vi "StopTask.vi"(8 "error in (no error)":errorcluster, 11 "NI_DAQmx(Linear) in":refnum<class "NI_DAQmx(Linear).lvclass">) -> (0 "error out":errorcluster, 3 "NI_DAQmx(Linear) out":refnum<class "NI_DAQmx(Linear).lvclass">)   [LabVIEW 2025, in "NI_DAQmx(Linear).lvclass"]
uses:
  NI_DAQmx(Linear).lvclass
  NI_DAQmx(Linear).lvclass/NI_DAQmx(Linear).ctl
  Read task.vi
  DAQ_Abstr/Task_Type/Linear_Task/Linear_Task/Linear_Task.lvclass
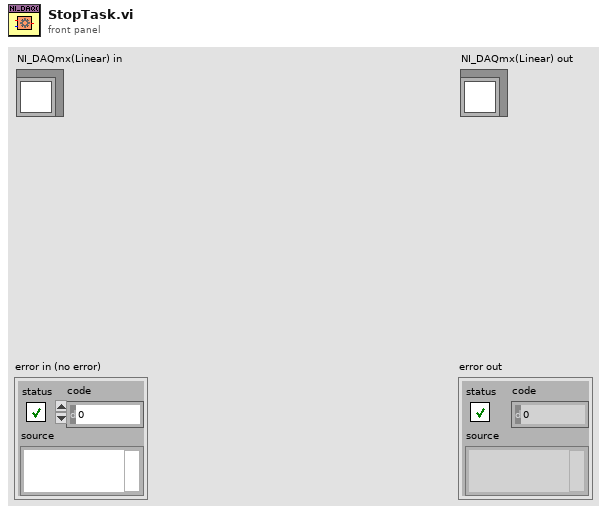
[diagram p1: front panel]
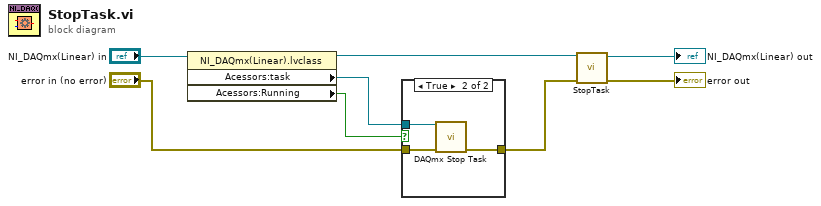
[diagram p0: block diagram]
diagram:
  n1 = property class="NI_DAQmx(Linear).lvclass"(reference="NI_DAQmx(Linear) in") -> (reference out=w3:refnum<class "NI_DAQmx(Linear).lvclass">, "Acessors:task"=w6:refnum<k21>, "Acessors:Running"=w5:bool)  [unwired: 1 in, 1 out]
  n2 = case shown="True" w5 {
    tunnel: w6 -> [_ w12]
    tunnel: [w9 w11] -> w1
    tunnel: "error in (no error)" -> [w9 w10]
    frame False {
    }
    frame True {
      n3 = call <vilib>:"DAQmx Stop Task.vi"("task/channels in"=w12, "error in"=w10) -> ("error out"=w11:errorcluster)  [unwired: 12 in, 1 out]
    }
  }
  n4 = call-parent "StopTask.vi"("error in (no error)"=w1, "Task_Abstr in"=w3) -> ("error out"=→"error out":errorcluster, "Task_Abstr out"=→"NI_DAQmx(Linear) out":refnum<class "NI_DAQmx(Linear).lvclass">)  [unwired: 8 in]
